vi "pythonwave.vi"(5 "Spreadsheet path":path=path "c:/Lab/waveform/MOTConf.csv", 7 "Script path":path=path "c:/Lab/waveform/script.py", 8 "error in (no error)":errorcluster, 10 "Loop number":i16, 11 "Update rate":i32=20000) -> (0 "error out":errorcluster, 2 "Waveforms":dbl[][](array[numeric])=[[11.0, 12.0, 13.0, 14.0], [21.0, 22.0, 23.0, 24.0]] format="%.2f")   [LabVIEW 2011]
uses:
  <userlib>/_OpenG.lib/labpython/labpython.llb/PYTHON Set String Data__ogtk.vi
  <userlib>/_OpenG.lib/labpython/labpython.llb/PYTHON Set Integer Data__ogtk.vi
  <userlib>/_OpenG.lib/labpython/labpython.llb/PYTHON Get Float Matrix__ogtk.vi
panel:
  out "Python script source code":string
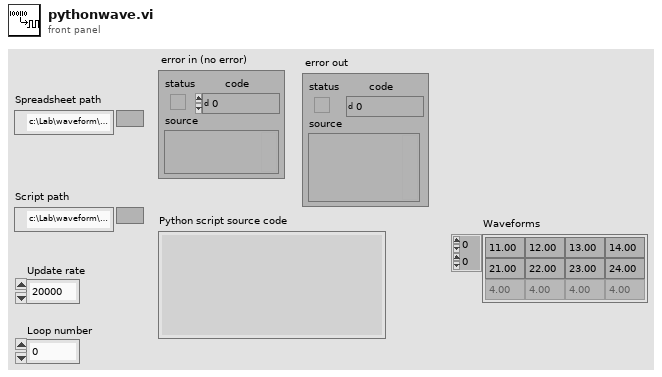
[diagram p1: front panel]
types:
  T1 = typedef "PYTHON Session Refnum__ogtk.ctl" = refnum<k1>
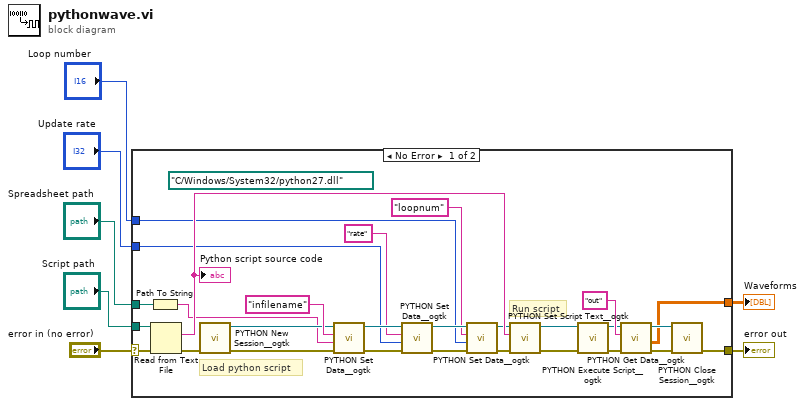
[diagram p0: block diagram]
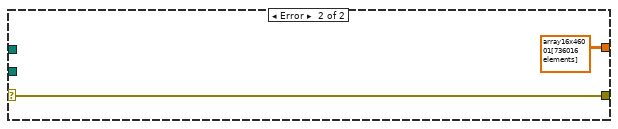
[diagram p2: hidden frame]
diagram:
  n1 = case shown="No Error" "error in (no error)" {
    selector: "error in (no error)" -> [w31 w36]
    tunnel: [w25 dbl[][] array16x46001[736016 elements] ("Waveforms 2")] -> w6
    tunnel: [w24 w36] -> w5
    tunnel: "Script path" -> [w23 _]
    tunnel: "Spreadsheet path" -> [w19 _]
    tunnel: "Update rate" -> [w15 _]
    tunnel: "Loop number" -> [w9 _]
    frame No Error {
      (unwired) path "C:/Windows/System32/python27.dll" ("Path")
      # "Load python script"
      # "Run script"
      n2 = Path To String(path=w19) -> (string=w18:string)
      n3 = Read from Text File(file (use dialog)=w23, error in=w31) -> (text=w32:string, error out=w35:errorcluster)  [unwired: 2 in, 2 out]
      "Python script source code" <- w32
      n4 = call <userlib>:"PYTHON New Session__ogtk.vi"("error in (no error)"=w35) -> ("error out"=w21:errorcluster, "Python Session"=w20:T1)  [unwired: 5 in]
      n5 = call-poly <userlib>:"PYTHON Set Data__ogtk.vi"("error in (no error)"=w21, "value"=w18, "variable name"="infilename", "Python Session in"=w20) -> ("error out"=w17:errorcluster, "Python Session out"=w16:T1)  [unwired: 2 in]
      n6 = call-poly <userlib>:"PYTHON Set Data__ogtk.vi"("error in (no error)"=w17, "value"=w15, "variable name"="rate", "Python Session in"=w16) -> ("error out"=w13:errorcluster, "Python Session out"=w11:T1)  [unwired: 2 in]
      n7 = call-poly <userlib>:"PYTHON Set Data__ogtk.vi"("error in (no error)"=w13, "value"=w9, "variable name"="loopnum", "Python Session in"=w11) -> ("error out"=w12:errorcluster, "Python Session out"=w10:T1)  [unwired: 2 in]
      n8 = call <userlib>:"PYTHON Set Script Text__ogtk.vi"("error in (no error)"=w12, "script text"=w32, "Python Session in"=w10) -> ("error out"=w33:errorcluster, "Python Session out"=w34:T1)  [unwired: 3 in]
      n9 = call <userlib>:"PYTHON Execute Script__ogtk.vi"("error in (no error)"=w33, "Python Session in"=w34) -> ("error out"=w27:errorcluster, "Python Session out"=w28:T1)  [unwired: 4 in]
      n10 = call-poly <userlib>:"PYTHON Get Data__ogtk.vi"("error in (no error)"=w27, "variable name"="out", "Python Session in"=w28) -> ("error out"=w26:errorcluster, "value"=w25:dbl[][], "Python Session out"=w30:T1)  [unwired: 2 in]
      n11 = call <userlib>:"PYTHON Close Session__ogtk.vi"("error in (no error)"=w26, "Python Session in"=w30) -> ("error out"=w24:errorcluster)  [unwired: 5 in]
    }
    frame Error {
    }
  }
  "Waveforms" <- w6
  "error out" <- w5
